vi "Testing_TimeCount.vi"() -> ()   [LabVIEW 2020]
uses:
  <vilib>/Analysis/NI_AALBase.lvlib
panel:
  in  "mean array size":i32=100 min=10 max=100000 step=10
  out "std":dbl format="%0.2f"
  out "mean elapsed T":dbl format="%0.2f"
  in  "Type of CountT VI":u16(ring) items=["Reentrant Clone", "Non-reentrant"]
  out "Elapsed time [ms]":u32
  in  "Suspend ms":u32=1 min=1 max=5000 step=1
  in  "stop":bool
  # "Testing capabilities of measuring of cycles timing"
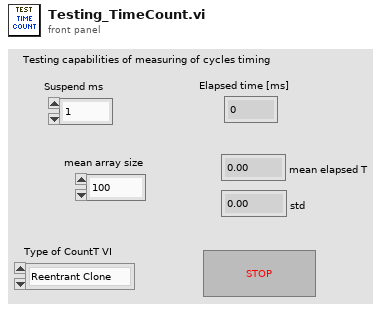
[diagram p1: front panel]
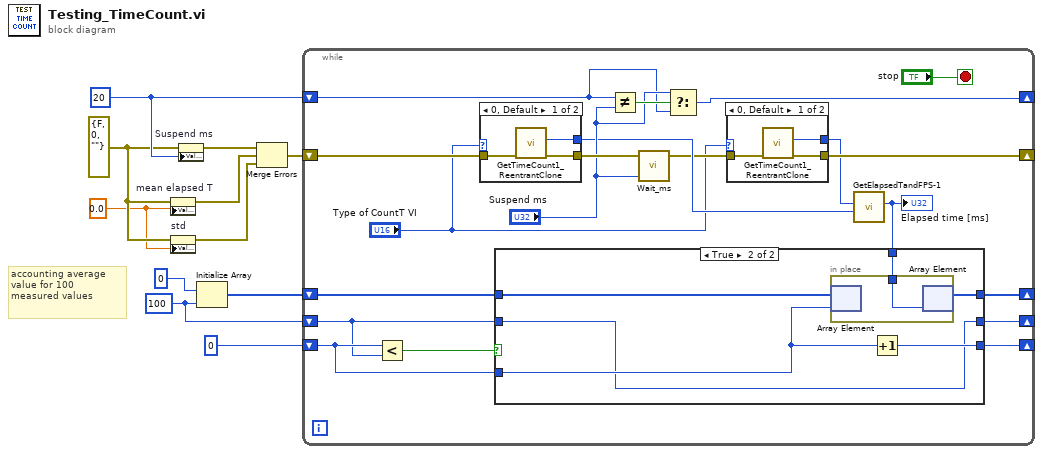
[diagram p0: block diagram]
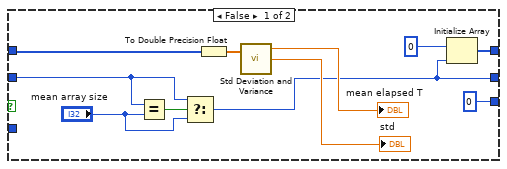
[diagram p2: hidden frame]
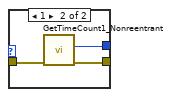
[diagram p3: hidden frame]
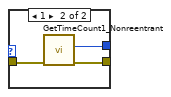
[diagram p4: hidden frame]
diagram:
  w1 = 0.0 ("mean elapsed T")
  w7 = 100 ("dimension size")
  w6 = errorcluster {"status"=FALSE, "code"=0, "source"=""} ("error IN")
  w11 = u32 20
  # "accounting average\nvalue for 100\nmeasured values"
  n1 = property on="mean elapsed T" class="DigNum (strict)"(error in=w6, "Value"=w1) -> (error out=w4:errorcluster)  [unwired: 1 in, 1 out]
  n2 = property on="std" class="DigNum (strict)"(error in=w6, "Value"=w1) -> (error out=w2:errorcluster)  [unwired: 1 in, 1 out]
  n3 = property on="Suspend ms" class="DigNum (strict)"(error in=w6, "Value"=w11) -> (error out=w5:errorcluster)  [unwired: 1 in, 1 out]
  n4 = Initialize Array(u32 0, w7) -> (w9:u32[])
  n5 = Merge Errors(w5, w4, w2) -> (w3:errorcluster)
  n6 = while {
    shift-right: [w25] -> _
    shift-left: w11 -> [w26]
    shift-right: [w22] -> _
    shift-left: w3 -> [w30]
    shift-right: [w15] -> _
    shift-left: w9 -> [w18]
    shift-right: [w14] -> _
    shift-left: 0 -> [w17]
    shift-right: [w12] -> _
    shift-left: w7 -> [w13]
    stop <- "stop" stop-if-true
    n7 = Less?(x=w17, y=w13) -> (x < y?=w19:bool)
    n8 = case shown="0, Default" "Type of CountT VI" {
      tunnel: w30 -> [w58 w61]
      tunnel: [w57 w60] -> w29
      tunnel: [w56 w59] -> w24
      frame 0, Default {
        n9 = call "GetTimeCount1_ReentrantClone.vi"("error IN"=w58) -> ("error OUT"=w57:errorcluster, "[OUT] Timer Count"=w56:u32)  [unwired: 9 in]
      }
      frame 1 {
        n10 = call "GetTimeCount1_Nonreentrant.vi"("error IN"=w61) -> ("error OUT"=w60:errorcluster, "[OUT] Timer Count"=w59:u32)  [unwired: 9 in]
      }
    }
    n11 = Not Equal?(x=w26, y="Suspend ms") -> (x != y?=w28:bool)
    n12 = call "Wait_ms.vi"("[IN] Suspend ms"="Suspend ms", "error IN"=w29) -> ("error OUT"=w23:errorcluster)  [unwired: 3 in]
    n13 = Select(t="Suspend ms", s=w28, f=w26) -> (s? t:f=w25:u32)
    n14 = case shown="0, Default" "Type of CountT VI" {
      tunnel: w23 -> [w52 w55]
      tunnel: [w51 w54] -> w22
      tunnel: [w50 w53] -> w21
      frame 0, Default {
        n15 = call "GetTimeCount1_ReentrantClone.vi"("error IN"=w52) -> ("error OUT"=w51:errorcluster, "[OUT] Timer Count"=w50:u32)  [unwired: 9 in]
      }
      frame 1 {
        n16 = call "GetTimeCount1_Nonreentrant.vi"("error IN"=w55) -> ("error OUT"=w54:errorcluster, "[OUT] Timer Count"=w53:u32)  [unwired: 9 in]
      }
    }
    n17 = call "GetElapsedTandFPS-1.vi"("[IN] Timer Count Before ALL [ms]"=w24, "[IN] Timer Count After ALL [ms]"=w21) -> ("[OUT] Elapsed time [ms]"=w16:u32)  [unwired: 3 in, 2 out]
    "Elapsed time [ms]" <- w16
    n18 = case shown="True" w19 {
      tunnel: w18 -> [w41 w48]
      tunnel: w17 -> [_ w45]
      tunnel: w16 -> [_ w47]
      tunnel: [w38 w46] -> w15
      tunnel: [0 w44] -> w14
      tunnel: w13 -> [w34 w43]
      tunnel: [w32 w43] -> w12
      frame False {
        n19 = Equal?(x=w34, y="mean array size") -> (x = y?=w35:bool)
        n20 = Select(t=w34, s=w35, f="mean array size") -> (s? t:f=w32:i32)
        n21 = To Double Precision Float(number=w41) -> (double precision float=w40:dbl[])
        n22 = call <vilib>:"Std Deviation and Variance.vi"("X"=w40) -> ("mean"=→"mean elapsed T":dbl, "standard deviation"=→"std":dbl)  [unwired: 1 in, 1 out]
        n23 = Initialize Array(u32 0, w32) -> (w38:u32[])
      }
      frame True {
        n24 = in-place {
          in-place-border: w47 -> [w49]
          n25 = in-place-array #1(w48, w45) -> ()  [unwired: 1 out]
          n26 = in-place-array #1(w49) -> (w46:u32[])  [unwired: 1 out]
        }
        n27 = Increment(x=w45) -> (x+1=w44:i32)
      }
    }
  }
